vi "SenderQueueDriver.vi"(0 "Queue Name":string, 5 "Enqueue Element":T1, 7 "Enqueue N Element":T1[](array[typedef]), 11 "error in (no error)":errorcluster, 13 "Enum":T2) -> (4 "Dequeue Element":T1, 15 "error out":errorcluster)   [LabVIEW 2023]
doc: "Used as queue driver to perform various queue operations like create queue, enqueue, dequeue, flush and close queue."
uses:
  TypeDefs/SenderQueueOperations.ctl
  TypeDefs/SenderStateDataCluster.ctl
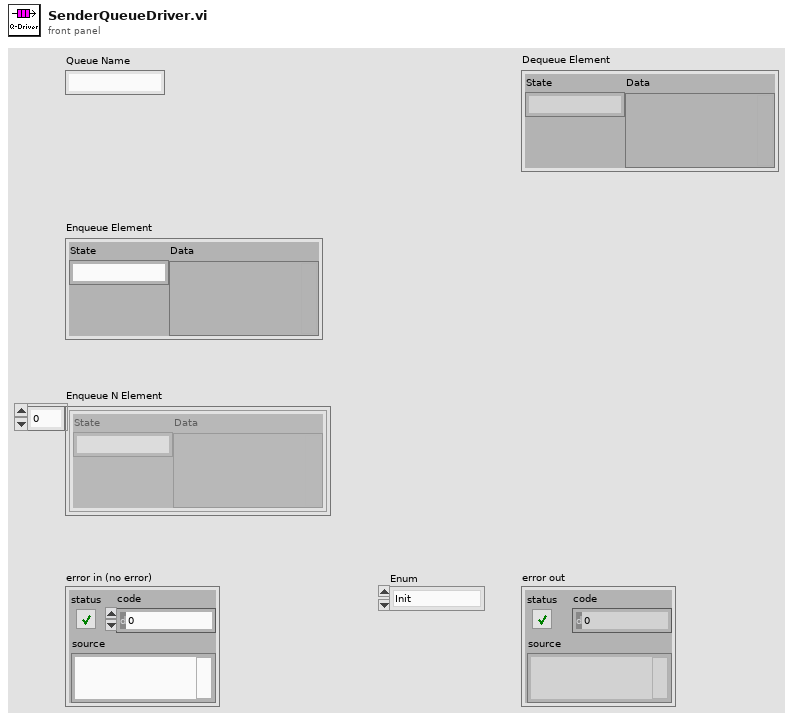
[diagram p1: front panel]
types:
  T1 = typedef "SenderStateDataCluster.ctl" = cluster{"State":string, "Data":variant}
  T2 = typedef "SenderQueueOperations.ctl" = enum16{"Init", "Enqueue", "Dequeue", "Enqueue N", "Flush", "Close", "Enqueue N Stack"}
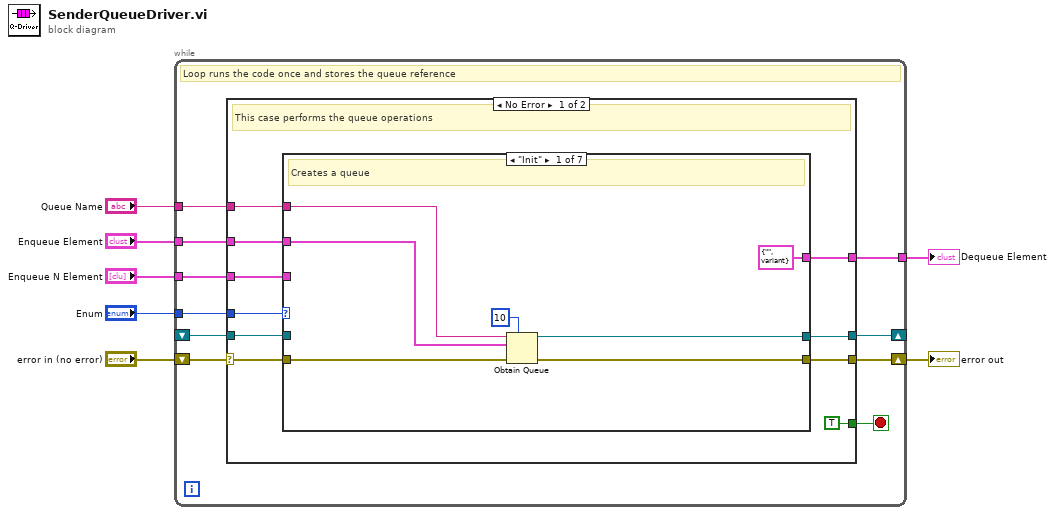
[diagram p0: block diagram]
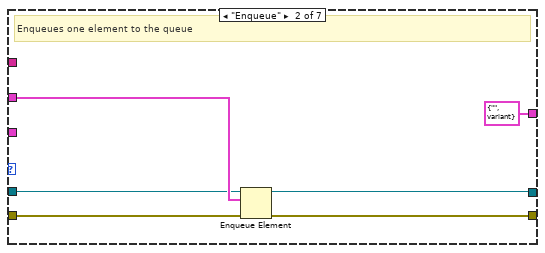
[diagram p2: hidden frame]
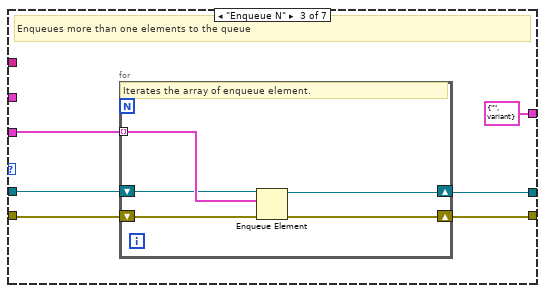
[diagram p3: hidden frame]
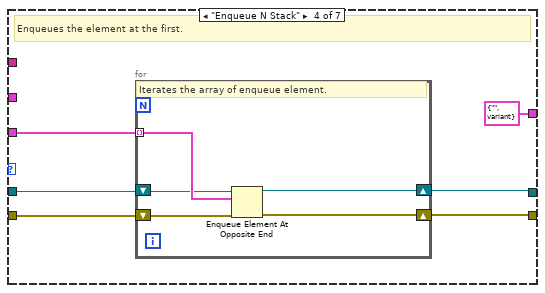
[diagram p4: hidden frame]
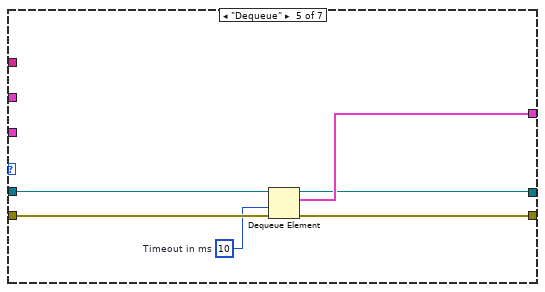
[diagram p5: hidden frame]
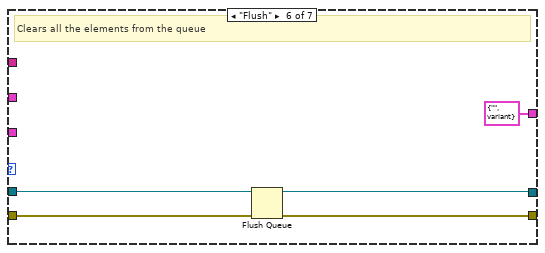
[diagram p6: hidden frame]
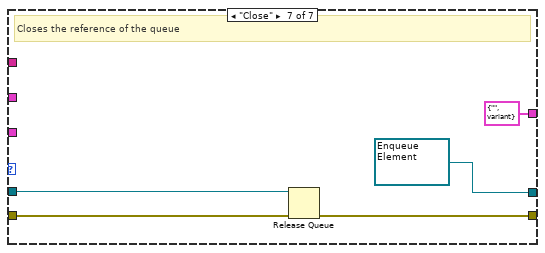
[diagram p7: hidden frame]
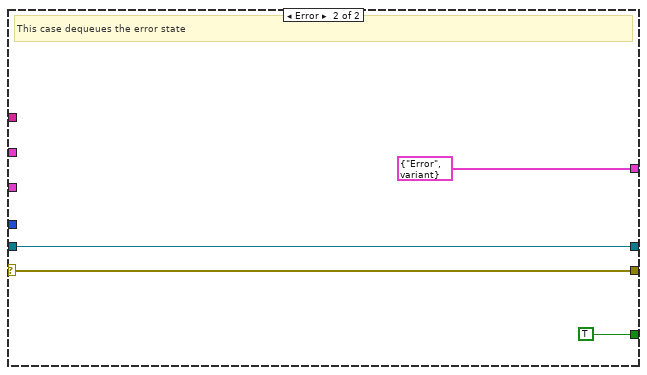
[diagram p8: hidden frame]
diagram:
  n1 = while {
    tunnel: "Queue Name" -> [w15]
    tunnel: "Enum" -> [w14]
    tunnel: "Enqueue N Element" -> [w13]
    tunnel: "Enqueue Element" -> [w12]
    tunnel: [w11] -> w1
    shift-right: [w10] -> _
    shift-left: _ -> [w9]
    shift-right: [w16] -> w6
    shift-left: "error in (no error)" -> [w17]
    stop <- w8 stop-if-true
    # "Loop runs the code once and stores the queue reference"
    n2 = case shown="No Error" w17 {
      selector: w17 -> [w26 w82]
      tunnel: w15 -> [w27 _]
      tunnel: [w25 w82] -> w16
      tunnel: w14 -> [w24 _]
      tunnel: w13 -> [w23 _]
      tunnel: w12 -> [w22 _]
      tunnel: [w21 T1 {"State"="Error", "Data"=variant} ("Enqueue Element")] -> w11
      tunnel: [w20 w80] -> w10
      tunnel: w9 -> [w19 w80]
      tunnel: [TRUE TRUE] -> w8
      frame No Error {
        # "This case performs the queue operations"
        n3 = case shown="\"Init\"" w24 {
          tunnel: w27 -> [w32 _ _ _ _ _ _]
          tunnel: w26 -> [w34 w40 w45 w57 w68 w73 w78]
          tunnel: [w33 w39 w44 w56 w67 w72 w77] -> w25
          tunnel: w23 -> [_ _ w46 w54 _ _ _]
          tunnel: w22 -> [w31 w38 _ _ _ _ _]
          tunnel: [T1 {"State"="", "Data"=variant} ("Enqueue Element") T1 {"State"="", "Data"=variant} ("Enqueue Element") T1 {"State"="", "Data"=variant} ("Enqueue Element") T1 {"State"="", "Data"=variant} ("Enqueue Element") w66 T1 {"State"="", "Data"=variant} ("Enqueue Element") T1 {"State"="", "Data"=variant} ("Enqueue Element")] -> w21
          tunnel: [w30 w36 w42 w53 w64 w70 refnum<queue> refnum ("queue out")] -> w20
          tunnel: w19 -> [_ w37 w43 w55 w65 w71 w76]
          frame "Init" {
            # "Creates a queue"
            n4 = Obtain Queue(max queue size (-1, unlimited)=10, name (unnamed)=w32, element data type=w31, error in (no error)=w34) -> (queue out=w30:refnum<queue>, error out=w33:errorcluster)  [unwired: 1 in, 1 out]
          }
          frame "Enqueue" {
            # "Enqueues one element to the queue"
            n5 = Enqueue Element(queue=w37, element=w38, error in (no error)=w40) -> (queue out=w36:refnum<queue>, error out=w39:errorcluster)  [unwired: 1 in, 1 out]
          }
          frame "Enqueue N" {
            # "Enqueues more than one elements to the queue"
            n6 = for {
              tunnel: w46 -> [w49] mode=indexing
              shift-right: [w48] -> w42
              shift-left: w43 -> [w47]
              shift-right: [w50] -> w44
              shift-left: w45 -> [w51]
              # "Iterates the array of enqueue element."
              n7 = Enqueue Element(queue=w47, element=w49, error in (no error)=w51) -> (queue out=w48:refnum<queue>, error out=w50:errorcluster)  [unwired: 1 in, 1 out]
            }
          }
          frame "Enqueue N Stack" {
            # "Enqueues the element at the first."
            n8 = for {
              shift-right: [w61] -> w56
              shift-left: w57 -> [w62]
              tunnel: w54 -> [w60] mode=indexing
              shift-right: [w58] -> w53
              shift-left: w55 -> [w59]
              # "Iterates the array of enqueue element."
              n9 = Enqueue Element At Opposite End(queue=w59, element=w60, error in (no error)=w62) -> (queue out=w58:refnum<queue>, error out=w61:errorcluster)  [unwired: 1 in, 1 out]
            }
          }
          frame "Dequeue" {
            w63 = 10  # Timeout in ms
            n10 = Dequeue Element(queue=w65, timeout in ms (-1)=w63, error in (no error)=w68) -> (queue out=w64:refnum<queue>, element=w66:T1, error out=w67:errorcluster)  [unwired: 1 out]
          }
          frame "Flush" {
            # "Clears all the elements from the queue"
            n11 = Flush Queue(queue=w71, error in (no error)=w73) -> (queue out=w70:refnum<queue>, error out=w72:errorcluster)  [unwired: 1 out]
          }
          frame "Close" {
            # "Closes the reference of the queue"
            n12 = Release Queue(queue=w76, error in (no error)=w78) -> (error out=w77:errorcluster)  [unwired: 1 in, 2 out]
          }
        }
      }
      frame Error {
        # "This case dequeues the error state"
      }
    }
  }
  "error out" <- w6
  "Dequeue Element" <- w1
